vi "bh3_get_unit_mac_address.vi"(8 "error in (no error)":errorcluster, 11 "bt connection ID in":refnum<k31>) -> (0 "error out":errorcluster, 2 "MAC Address":string, 3 "bt connection ID out":refnum<k31>)   [LabVIEW 2013]
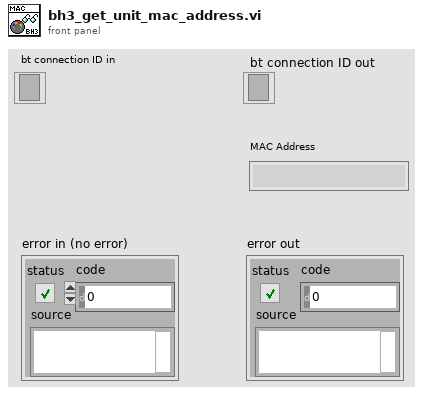
[diagram p1: front panel]
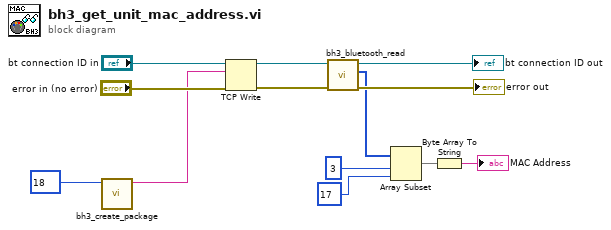
[diagram p0: block diagram]
diagram:
  n1 = call "bh3_create_package.vi"("msg_ID"=u8 18) -> ("package string"=w10:string)  [unwired: 9 in, 1 out]
  n2 = TCP Write(connection ID="bt connection ID in", data in=w10, error in (no error)="error in (no error)") -> (connection ID out=w6:refnum<k31>, error out=w9:errorcluster)  [unwired: 1 in, 1 out]
  n3 = call "bh3_bluetooth_read.vi"("error in (no error)"=w9, "bt connection ID in"=w6) -> ("error out"=→"error out":errorcluster, "response byte array"=w5:u8[], "bt connection ID out"=→"bt connection ID out":refnum<k31>)  [unwired: 7 in]
  n4 = Array Subset(array=w5, index=3, length=17 ("index")) -> (w2:u8[])
  n5 = Byte Array To String(unsigned byte array=w2) -> (string=→"MAC Address":string)
